vi "Part 1.vi"(11 "Input":string) -> (3 "Output":i64)   [LabVIEW 2021]
uses:
  c234f0d4-0e6c-49fd-9763-9d7dce579a2e.vi
  <userlib>/_OpenG.lib/array/array.llb/Search 1D Array (String)__ogtk.vi
  <userlib>/_OpenG.lib/array/array.llb/Index 1D Array Elements (String)__ogtk.vi
panel:
  out "map in":map{string, string[]}(c390)
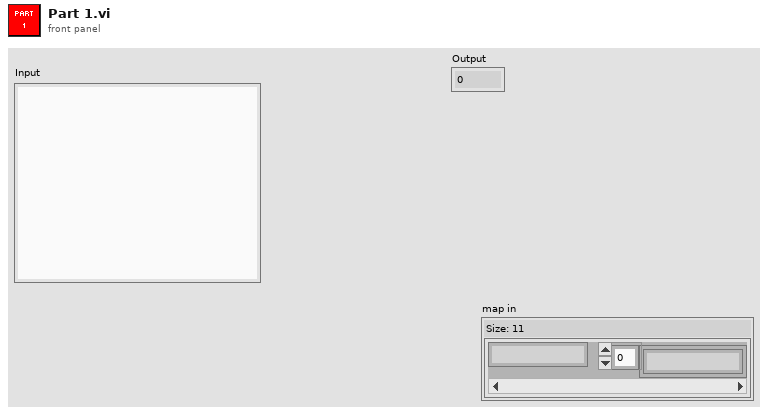
[diagram p1: front panel]
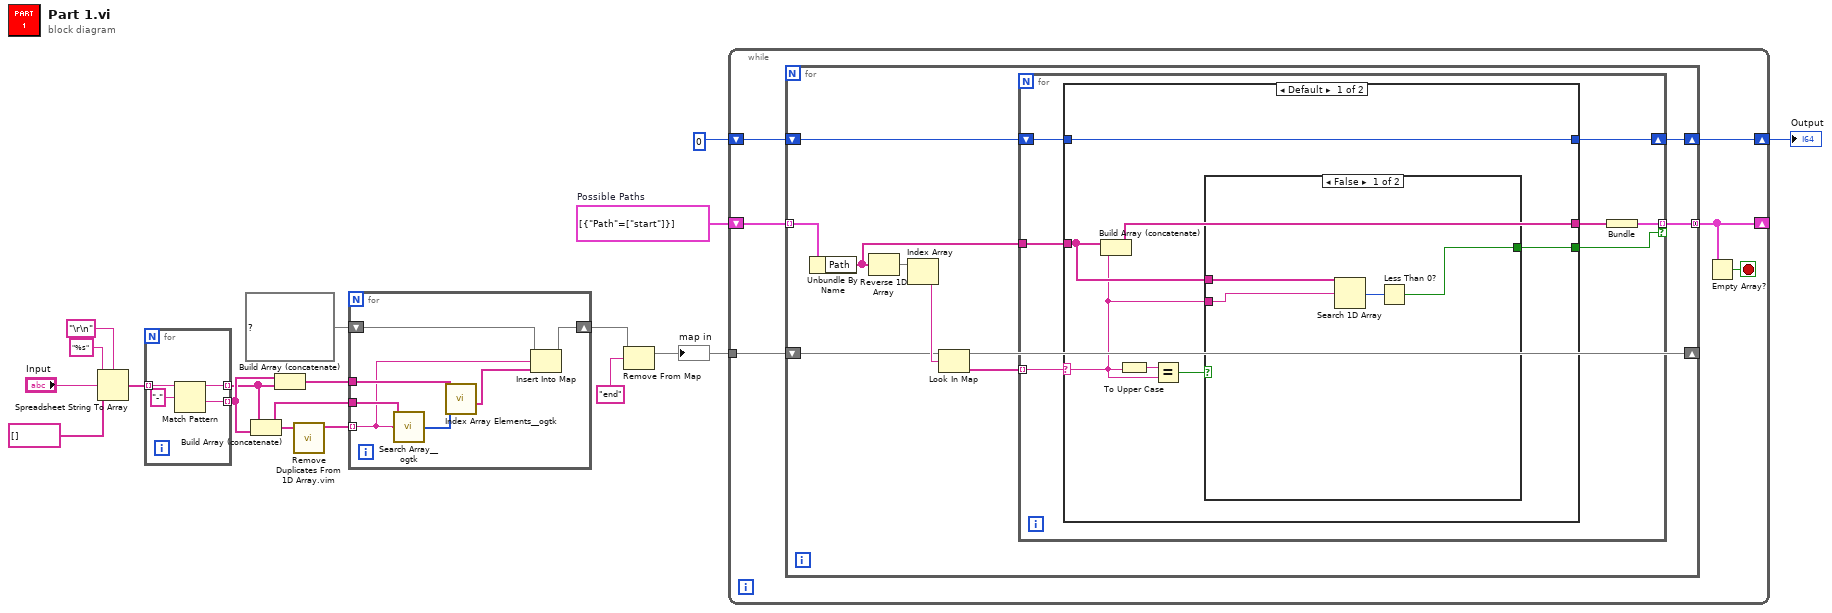
[diagram p0: block diagram]
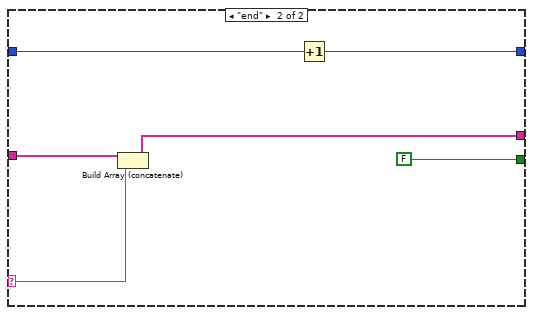
[diagram p3: hidden frame]
diagram:
  w4 = cluster{"Path":string[]}[] [{"Path"=["start"]}]  # Possible Paths
  n1 = Spreadsheet String To Array(delimiter (Tab)="\r\n", format string="%s", spreadsheet string="Input", array type (2D Dbl)=string[] []) -> (array=w13:string[])
  n2 = for {
    tunnel: w13 -> [w21] mode=indexing
    tunnel: [w19] -> w10 mode=indexing
    tunnel: [w18] -> w11 mode=indexing
    n3 = Match Pattern(string=w21, regular expression="-") -> (before substring=w19:string, after substring=w18:string)  [unwired: 1 in, 2 out]
  }
  n4 = Build Array (concatenate)(w10, w11) -> (w9:string[])
  n5 = Build Array (concatenate)(w11, w10) -> (w8:string[])
  n6 = call "Remove Duplicates From 1D Array.vim"("array"=w9) -> ("array with duplicates removed"=w12:string[])  [unwired: 10 in]
  n7 = for {
    tunnel: w12 -> [w25] mode=indexing
    tunnel: w9 -> [w28]
    tunnel: w8 -> [w27]
    shift-right: [w22] -> w6
    shift-left: map{string, string[]} {} ("map in") -> [w23]
    n8 = call-poly <userlib>:"Search Array__ogtk.vi"("Array"=w28, "Element Data"=w25) -> ("Indices of Elements"=w26:i32[])  [unwired: 7 in]
    n9 = call-poly <userlib>:"Index Array Elements__ogtk.vi"("indices"=w26, "array"=w27) -> ("elements"=w24:string[])  [unwired: 9 in]
    n10 = Insert Into Map(map in=w23, key=w25, value=w24) -> (map out=w22:map{string, string[]})  [unwired: 2 out]
  }
  n11 = Remove From Map(10:"end" ("key"), 11:w6) -> (3:w1:map{string, string[]})  [unwired: 2 out]
  "map in" <- w1
  n12 = while {
    shift-right: [w29] -> _
    shift-left: w4 -> [w33]
    shift-right: [w31] -> w2
    shift-left: i64 0 -> [w32]
    tunnel: w1 -> [w30]
    stop <- w34 stop-if-true
    n13 = for {
      tunnel: w33 -> [w36] mode=indexing
      shift-right: [w39] -> w31
      shift-left: w32 -> [w40]
      shift-right: [w41] -> _
      shift-left: w30 -> [w41]
      tunnel: [w35] -> w29 mode=concatenating
      n14 = Unbundle By Name(w36) -> ("Path"=w37:string[])
      n15 = Reverse 1D Array(array=w37) -> (reversed array=w43:string[])
      n16 = Index Array(array=w43) -> (element=w42:string)  [unwired: 1 in]
      n17 = Look In Map(map=w41, key=w42) -> (value=w38:string[])  [unwired: 1 in, 1 out]
      n18 = for {
        shift-right: [w48] -> w39
        shift-left: w40 -> [w49]
        tunnel: w38 -> [w50] mode=indexing
        tunnel: w37 -> [w45]
        tunnel: [w47] -> w35 mode=indexing if=w46
        n19 = case shown="Default" w50 {
          selector: w50 -> [w51 w64]
          tunnel: w49 -> [w57 w68]
          tunnel: [w57 w67] -> w48
          tunnel: [w53 FALSE] -> w46
          tunnel: w45 -> [w52 w65]
          tunnel: [w56 w63] -> w44
          frame Default {
            n20 = Build Array (concatenate)(w52, w51) -> (w56:string[])
            n21 = To Upper Case(1:w51) -> (0:w55:string)
            n22 = Equal?(x=w55, y=w51) -> (x = y?=w54:bool)
            n23 = case shown="False" w54 {
              selector: w54 -> [_ w62]
              tunnel: [w59 w62] -> w53
              tunnel: w52 -> [w58 _]
              tunnel: w51 -> [w61 _]
              frame False {
                n24 = Search 1D Array(1D array=w58, element=w61) -> (index of element=w60:i32)  [unwired: 1 in]
                n25 = Less Than 0?(x=w60) -> (x < 0?=w59:bool)
              }
              frame True {
              }
            }
          }
          frame "end" {
            n26 = Build Array (concatenate)(w65, w64) -> (w63:string[])
            n27 = Increment(x=w68) -> (x+1=w67:i64)
          }
        }
        n28 = Bundle(w44) -> (w47:cluster{string[]})  [unwired: 1 in]
      }
    }
    n29 = Empty Array?(array=w29) -> (empty?=w34:bool)
  }
  "Output" <- w2
